vi "Sequence.vi"(11 "Nodes":refnum<class "bt_Node.lvclass">[](array[class])) -> (3 "Node":refnum<class "bt_Node.lvclass">)   [LabVIEW 2021, in "BT.lvlib"]
uses:
  BT.lvlib
  Support/Nodes/abs_Node/bt_Node.lvclass
  Support/Nodes/Composites/Sequence/bt_Sequence.lvclass
  C:/Users/Tim/Documents/GitHub/LV_Behaviour_Tree/Source/Support/Nodes/Composites/abs_Composite/bt_Composite.lvclass
  C:/Users/Tim/Documents/GitHub/LV_Behaviour_Tree/Source/Support/Nodes/abs_Node/bt_Node.lvclass
  Support/Nodes/Composites/abs_Composite/bt_Composite.lvclass/bt_Composite.ctl
  Support/Nodes/Composites/abs_Composite/Properties/Write Nodes.vi
  C:/Users/Tim/Documents/GitHub/LV_Behaviour_Tree/Source/Support/Nodes/Composites/Sequence/bt_Sequence.lvclass
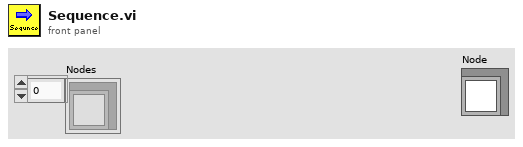
[diagram p1: front panel]
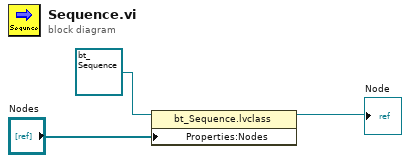
[diagram p0: block diagram]
diagram:
  n1 = property class="bt_Sequence.lvclass"(reference=refnum<class "bt_Sequence.lvclass"> refnum ("BT.lvlib:Sequence.lvclass"), "Properties:Nodes"="Nodes") -> (reference out=→"Node":refnum<class "bt_Sequence.lvclass">)  [unwired: 1 in, 1 out]
